vi "CSM - Query CSM VI Ref By API String.vi"(6 "Response Timeout(5000ms)":i32=5000, 7 "Current Module(\"\" to generate a ID)":string, 8 "Error In (no error)":errorcluster, 9 "Target Module":string="A") -> (0 "error out":errorcluster, 3 "CSM VI Ref":refnum<vi>)   [LabVIEW 2017, in "API String Arguments Support.lvlib"]
uses:
  API String Arguments Support.lvlib
  <userlib>/_NEVSTOP/Communicable State Machine(CSM)/_Support/Priority Queue/Priority Queue.lvclass/Priority Queue.ctl
  <userlib>/_NEVSTOP/Communicable State Machine(CSM)/Utility/Build Error Cluster.vi
  <userlib>/_NEVSTOP/Communicable State Machine(CSM)/_Support/Process/CSMP-Sync Call.vi
  <userlib>/_NEVSTOP/Communicable State Machine(CSM)/Utility/uuid.vi
  <userlib>/_NEVSTOP/Communicable State Machine(CSM)/Utility/Trim Both Whitespace.vi
  <userlib>/_NEVSTOP/Communicable State Machine(CSM)/_Support/CSMQ/_CSMObj-Message Check.vi
  <userlib>/_NEVSTOP/Communicable State Machine(CSM)/_Support/CSMQ/_CSMObj-Enqueue Cross-Module Message.vi
  <userlib>/_NEVSTOP/Communicable State Machine(CSM)/_Support/CSMQ/_CSMOFGV Get.vi
  <userlib>/_NEVSTOP/Communicable State Machine(CSM)/_Support/Priority Queue/Enqueue Element.vi
  <userlib>/_NEVSTOP/Communicable State Machine(CSM)/_Support/CSMQ/_CSMOFGV.vi
  <userlib>/_NEVSTOP/Communicable State Machine(CSM)/Communicable State Machine.lvlib
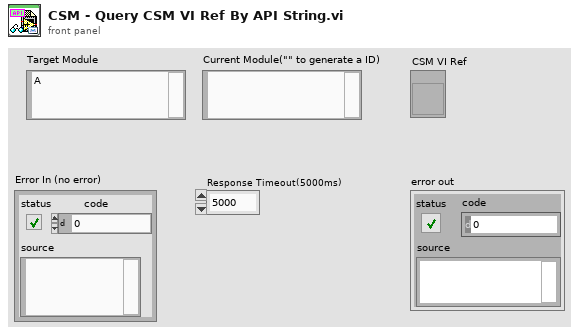
[diagram p1: front panel]
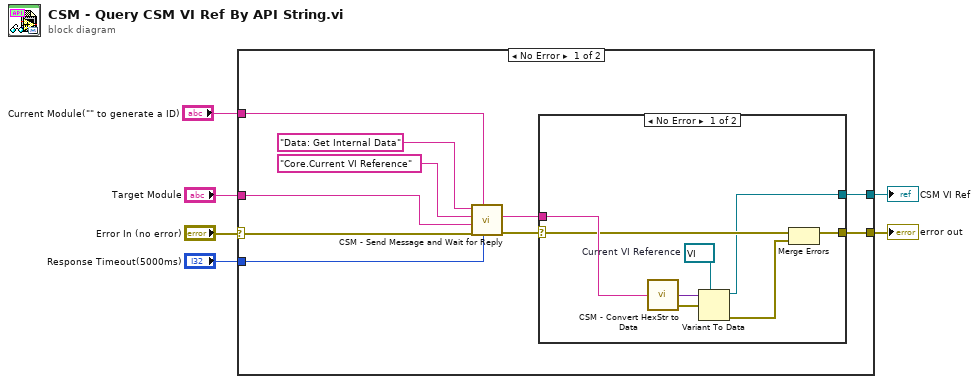
[diagram p0: block diagram]
diagram:
  n1 = case shown="No Error" "Error In (no error)" {
    selector: "Error In (no error)" -> [w11 w26]
    tunnel: "Response Timeout(5000ms)" -> [w15 _]
    tunnel: [w12 w26] -> w5
    tunnel: [w9 _] -> w3
    tunnel: "Target Module" -> [w8 _]
    tunnel: "Current Module(\"\" to generate a ID)" -> [w7 _]
    frame No Error {
      n2 = call <userlib>:"CSM - Send Message and Wait for Reply.vi"("Response Timeout(5000ms)"=w15, "Current Module(\"\" to generate a ID)"=w7, "Error In (no error)"=w11, "Target Module"=w8, "Arguments (\"\")"="Core.Current VI Reference" ("Name(\"\" to use uuid)"), "State"="Data: Get Internal Data") -> ("error out"=w13:errorcluster, "Arguments"=w14:string)  [unwired: 3 in, 1 out]
      n3 = case shown="No Error" w13 {
        selector: w13 -> [w19 w25]
        tunnel: w14 -> [w24 _]
        tunnel: [w20 w25] -> w12
        tunnel: [w17 _] -> w9
        frame No Error {
          w21 = refnum<vi> refnum  # Current VI Reference
          n4 = call <userlib>:"CSM - Convert HexStr to Data.vi"("HEX String"=w24) -> ("Variant"=w22:variant, "error out"=w23:errorcluster)  [unwired: 7 in]
          n5 = Variant To Data(error in=w23, type=w21, Variant=w22) -> (data=w17:refnum<vi>, error out=w18:errorcluster)
          n6 = Merge Errors(w19, w18) -> (w20:errorcluster)
        }
        frame Error {
        }
      }
    }
    frame Error {
    }
  }
  "error out" <- w5
  "CSM VI Ref" <- w3
